vi "format display.vi"(6 "Channel":i32(slide)=1 min=0 max=7 step=1 scale=0.0..7.0, 8 "error in (no error)":errorcluster, 9 "Display":enum16{"X and Y", "R and Theta"}(ring), 10 "Results (X,Y,R,Theta)":dbl[][](array[numeric])) -> (0 "error out":errorcluster, 1 "Array 2":cluster{dbl[], dbl[]}[](array[cluster]), 2 "Y/Theta Array":waveform(dbl)[](array[waveform]), 3 "X/R Array":waveform(dbl)[](array[waveform]), 5 "Y/R":dbl, 7 "X/R":dbl)   [LabVIEW 2016, in "Instrument.Lockin.lvclass"]
uses:
  Instrument.Lockin.lvclass
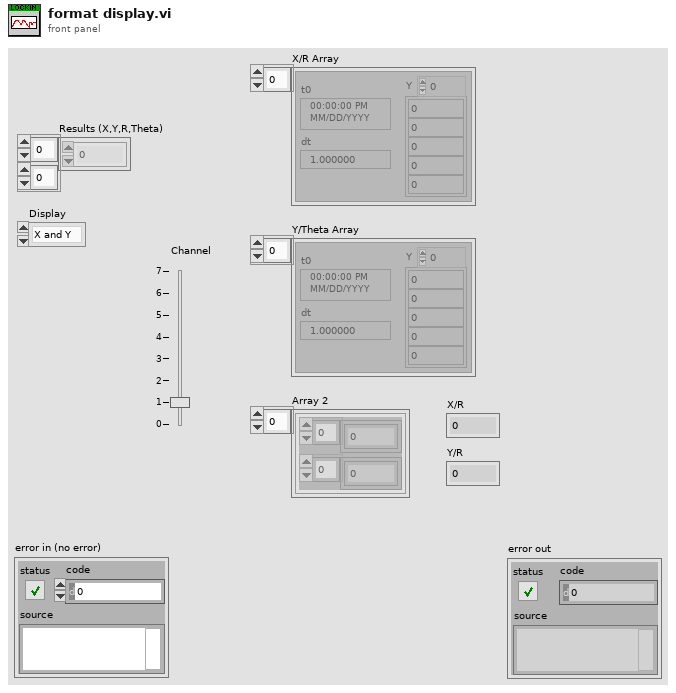
[diagram p1: front panel]
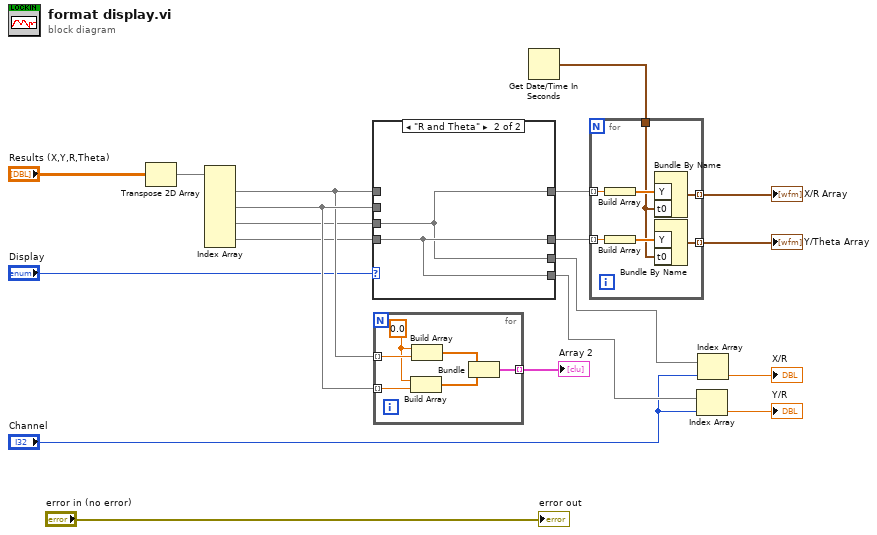
[diagram p0: block diagram]
diagram:
  n1 = Transpose 2D Array(2D array="Results (X,Y,R,Theta)") -> (transposed array=w10:dbl[][])
  n2 = Index Array(array=w10) -> (element #1=w16:dbl[], element #2=w17:dbl[], element #3=w13:dbl[], element #4=w14:dbl[])  [unwired: 8 in]
  n3 = case shown="\"R and Theta\"" "Display" {
    tunnel: w16 -> [w20 _]
    tunnel: [w20 w22] -> w9
    tunnel: w17 -> [w21 _]
    tunnel: [w21 w23] -> w8
    tunnel: w13 -> [_ w22]
    tunnel: w14 -> [_ w23]
    tunnel: [w21 w23] -> w6
    tunnel: [w20 w22] -> w7
    frame "X and Y", Default {
    }
    frame "R and Theta" {
    }
  }
  n4 = for {
    tunnel: w16 -> [w29] mode=indexing
    tunnel: w17 -> [w28] mode=indexing
    tunnel: [w24] -> w18 mode=indexing
    w27 = 0.0
    n5 = Build Array(w27, w28) -> (w25:dbl[])
    n6 = Build Array(w27, w29) -> (w26:dbl[])
    n7 = Bundle(w26, w25) -> (w24:cluster{dbl[], dbl[]})  [unwired: 1 in]
  }
  "Array 2" <- w18
  n8 = Get Date/Time In Seconds() -> (seconds since 1Jan1904=w2:timestamp)
  n9 = for {
    tunnel: w9 -> [w36] mode=indexing
    tunnel: w8 -> [w35] mode=indexing
    tunnel: [w34] -> w15 mode=indexing
    tunnel: [w33] -> w19 mode=indexing
    tunnel: w2 -> [w30]
    n10 = Build Array(w36) -> (w32:dbl[])
    n11 = Build Array(w35) -> (w31:dbl[])
    n12 = Bundle By Name("Y"=w32, "t0"=w30) -> (w34:waveform(dbl))  [unwired: 1 in]
    n13 = Bundle By Name("Y"=w31, "t0"=w30) -> (w33:waveform(dbl))  [unwired: 1 in]
  }
  "Y/Theta Array" <- w19
  "X/R Array" <- w15
  n14 = Index Array(array=w6, index="Channel") -> (element=→"Y/R":dbl)
  n15 = Index Array(array=w7, index="Channel") -> (element=→"X/R":dbl)
  "error out" <- "error in (no error)"
